vi "tester.vi"   [LabVIEW 2019]
types:
  T1 = enum16{"open", "replace", "create", "open or create", "replace or create", "replace or create with confirmation"}
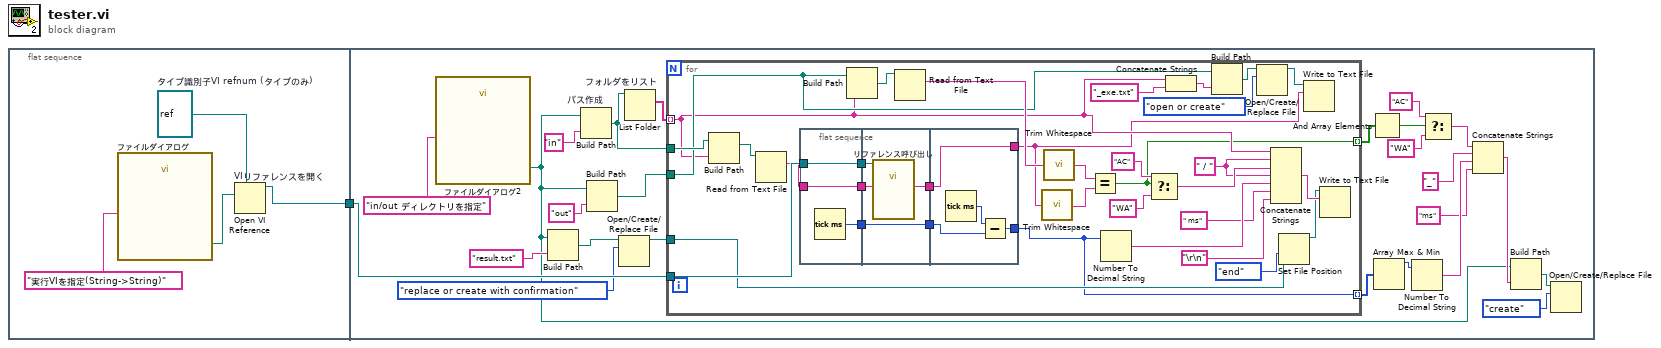
[diagram p0: block diagram]
diagram:
  n1 = flat-sequence {
    tunnel: [w5] -> w1
    tunnel: w1 -> [w27]
    frame #0 {
      w4 = refnum<vi> refnum  # タイプ識別子VI refnum (タイプのみ)
      n2 = call "ファイルダイアログ"("prompt"="実行VIを指定(String->String)") -> ("selected path"=w3:path)  [unwired: 11 in, 3 out]
      n3 = Open VI Reference "VIリファレンスを開く"(type specifier VI Refnum (for type only)=w4, vi path=w3) -> (vi reference=w5:refnum<vi>)  [unwired: 4 in, 1 out]
    }
    frame #1 {
      n4 = call "ファイルダイアログ2"("prompt"="in/out ディレクトリを指定") -> ("selected path"=w9:path)  [unwired: 11 in, 3 out]
      n5 = Build Path(base path=w9, name or relative path="result.txt") -> (appended path=w22:path)
      n6 = Build Path "パス作成"(base path=w9, name or relative path="in") -> (appended path=w26:path)
      n7 = Build Path ("パス作成")(base path=w9, name or relative path="out") -> (appended path=w25:path)
      n8 = Open/Create/Replace File(file path (use dialog)=w22, operation (0:open)=T1."replace or create with confirmation" ("操作 (0:open)")) -> (refnum out=w21:refnum<file>)  [unwired: 4 in, 2 out]
      n9 = List Folder "フォルダをリスト"(path=w26) -> (filenames=w28:string[])  [unwired: 3 in, 3 out]
      n10 = for {
        tunnel: w27 -> [w64]
        tunnel: w28 -> [w38] mode=indexing
        tunnel: w26 -> [w58]
        tunnel: w25 -> [w39]
        tunnel: w21 -> [w43]
        tunnel: [w40] -> w20 mode=indexing
        tunnel: [w34] -> w18 mode=indexing
        w47 = " / "
        n11 = Build Path ("パス作成")(base path=w58, name or relative path=w38) -> (appended path=w61:path)
        n12 = Read from Text File(file (use dialog)=w61) -> (text=w63:string)  [unwired: 3 in, 3 out]
        n13 = flat-sequence {
          tunnel: w63 -> [w66]
          tunnel: w64 -> [w67]
          tunnel: [w67] -> w54
          tunnel: [w66] -> w53
          tunnel: [w65] -> w51
          tunnel: [w69] -> w55
          tunnel: w54 -> [w71]
          tunnel: w53 -> [w70]
          tunnel: [w68] -> w52
          tunnel: w51 -> [w68]
          tunnel: [w75] -> w31
          tunnel: w55 -> [w75]
          tunnel: w52 -> [w73]
          tunnel: [w74] -> w40
          frame #0 {
            n14 = Tick Count (ms)() -> (millisecond timer value=w65:u32)
          }
          frame #1 {
            n15 = call-by-ref "リファレンス呼び出し"(reference=w71, "文字列入力"=w70) -> ("文字列出力"=w69:string)  [unwired: 11 in, 2 out]
          }
          frame #2 {
            n16 = Tick Count (ms)() -> (millisecond timer value=w72:u32)
            n17 = Subtract(x=w72, y=w73) -> (x-y=w74:u32)
          }
        }
        n18 = Build Path ("パス作成")(base path=w39, name or relative path=w38) -> (appended path=w56:path)
        n19 = Read from Text File(file (use dialog)=w56) -> (text=w62:string)  [unwired: 3 in, 3 out]
        n20 = call <vilib>:"Trim Whitespace.vi"("string"=w31) -> ("trimmed string"=w59:string)  [unwired: 1 in]
        n21 = call <vilib>:"Trim Whitespace.vi"("string"=w62) -> ("trimmed string"=w60:string)  [unwired: 1 in]
        n22 = Equal?(x=w60, y=w59) -> (x = y?=w34:bool)
        n23 = Number To Decimal String(number=w40) -> (decimal integer string=w46:string)  [unwired: 1 in]
        n24 = Select(t="AC", s=w34, f="WA") -> (s? t:f=w48:string)
        n25 = Concatenate Strings(w38, "_exe.txt") -> (w36:string)
        n26 = Build Path(base path=w39, name or relative path=w36) -> (appended path=w33:path)
        n27 = Open/Create/Replace File(file path (use dialog)=w33, operation (0:open)=T1."open or create" ("操作 (0:open)")) -> (refnum out=w32:refnum<file>)  [unwired: 4 in, 2 out]
        n28 = Concatenate Strings(w38, w47, w48, w47, w46, " ms", "\r\n") -> (w57:string)
        n29 = Set File Position(refnum=w43, from (0:start)=enum16{"start", "end", "current"}."end" ("基点 (0:start)")) -> (refnum out=w41:refnum<file>)  [unwired: 2 in, 1 out]
        n30 = Write to Text File(file (use dialog)=w32, text=w31) -> ()  [unwired: 2 in, 3 out]
        n31 = Write to Text File(file (use dialog)=w41, text=w57) -> ()  [unwired: 2 in, 3 out]
      }
      n32 = And Array Elements(Boolean array=w18) -> (logical AND=w17:bool)
      n33 = Array Max & Min(array=w20) -> (max value=w19:u32)  [unwired: 3 out]
      n34 = Number To Decimal String(number=w19) -> (decimal integer string=w12:string)  [unwired: 1 in]
      n35 = Select(t="AC", s=w17, f="WA") -> (s? t:f=w14:string)
      n36 = Concatenate Strings(w14, "_", w12, "ms") -> (w10:string)
      n37 = Build Path(base path=w9, name or relative path=w10) -> (appended path=w8:path)
      n38 = Open/Create/Replace File(file path (use dialog)=w8, operation (0:open)=T1."create" ("操作 (0:open)")) -> ()  [unwired: 4 in, 3 out]
    }
  }
